vi "Ramp_Staircase.vi"(5 "# Steps (10)":i32=10, 6 "Step Height (1) / nm":dbl=1.0, 7 "Error In":errorcluster, 8 "Ramp Time (1) / s":dbl=1.0, 10 "Acquisition Rate (20000) / Hz":dbl=20000.0) -> (0 "Error Out":errorcluster, 3 "Piezo Out / nm":dbl[](array[numeric]))   [LabVIEW 2023]
panel:
  out "Waveform Graph":dbl[](graph)
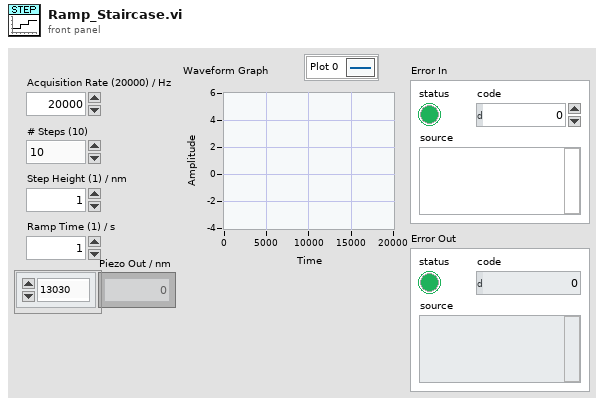
[diagram p1: front panel]
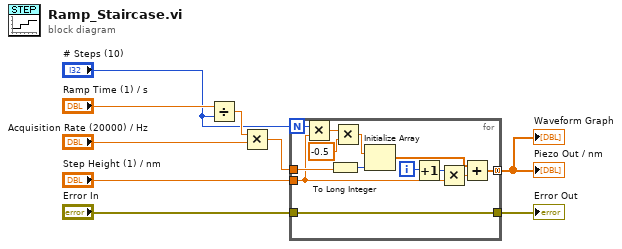
[diagram p0: block diagram]
diagram:
  n1 = Divide(x="Ramp Time (1) / s", y="# Steps (10)") -> (x/y=w3:dbl)
  n2 = Multiply(x=w3, y="Acquisition Rate (20000) / Hz") -> (x*y=w2:dbl)
  n3 = for {
    N: "# Steps (10)" -> [w14]
    tunnel: "Error In" -> [w22]
    tunnel: [w22] -> w8
    tunnel: "Step Height (1) / nm" -> [w13]
    tunnel: [w17] -> w5 mode=concatenating
    tunnel: w2 -> [w21]
    i -> [w16]
    n4 = Multiply(x=w14, y=w13) -> (x*y=w12:dbl)
    n5 = To Long Integer(number=w21) -> (32bit integer=w20:i32)
    n6 = Multiply(x=w12, y=-0.5) -> (x*y=w10:dbl)
    n7 = Initialize Array(w10, w20) -> (w19:dbl[])
    n8 = Increment(x=w16) -> (x+1=w15:i32)
    n9 = Multiply(x=w15, y=w13) -> (x*y=w18:dbl)
    n10 = Add(x=w19, y=w18) -> (x+y=w17:dbl[])
  }
  "Waveform Graph" <- w5
  "Piezo Out / nm" <- w5
  "Error Out" <- w8
